vi "GlobalDefaultFolderPath.vi"() -> ()   [LabVIEW 2018]
panel:
  out "String":string
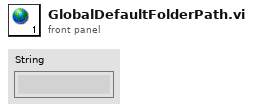
[diagram p1: front panel]
diagram:
